vi "OP400ZP_SendToBddOP100ZENPlus.vi"(8 "errin":errorcluster, 11 "data in":string[](array[string])=["", "2022-08-23 16:19:54.000000", "0", "test base", "1.1", "2", "3", "4", "5", "6", "7", "8", "9", "10", "11", "12", "13", "14", "15", "16", "17", "18", "19", "20", "21", "22", "23", "24", "25", "26", "27", "1", "MOI", "28"]) -> (0 "error out":errorcluster, 3 "Chaîne":string)   [LabVIEW 2020]
uses:
  <vilib>/addons/database/Connection.llb/DB Tools Open Connec (String).vi
  <vilib>/addons/database/Connection.llb/Conn Execute.vi
  <vilib>/addons/database/Recordset.llb/Rec Destroy - Connection.vi
  <vilib>/addons/database/NI_Database_API.lvlib
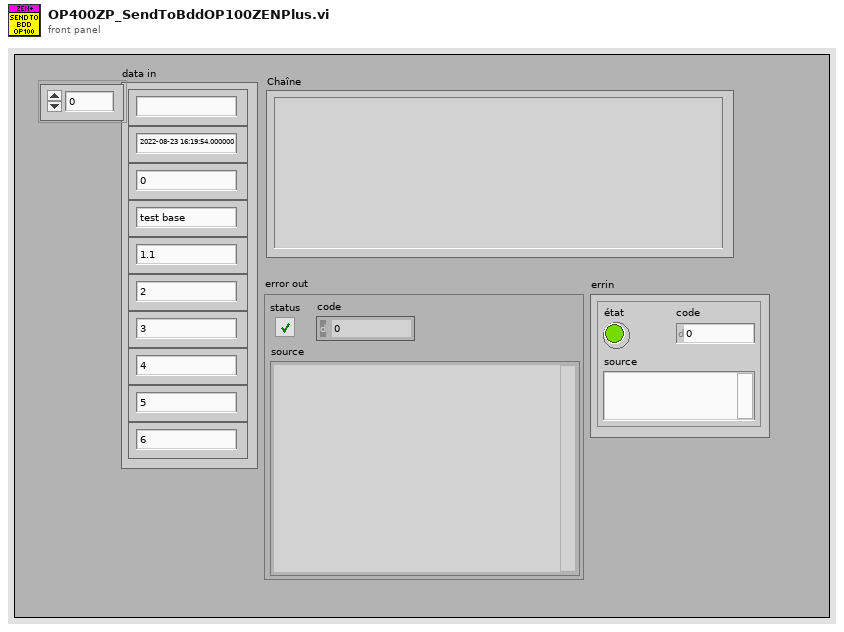
[diagram p1: front panel]
types:
  T1 = typedef "NI_Database_API.lvlib/Conn ObjectReference.ctl" = refnum<k1>
  T2 = typedef "NI_Database_API.lvlib/Rec ObjectReference.ctl" = refnum<k1>
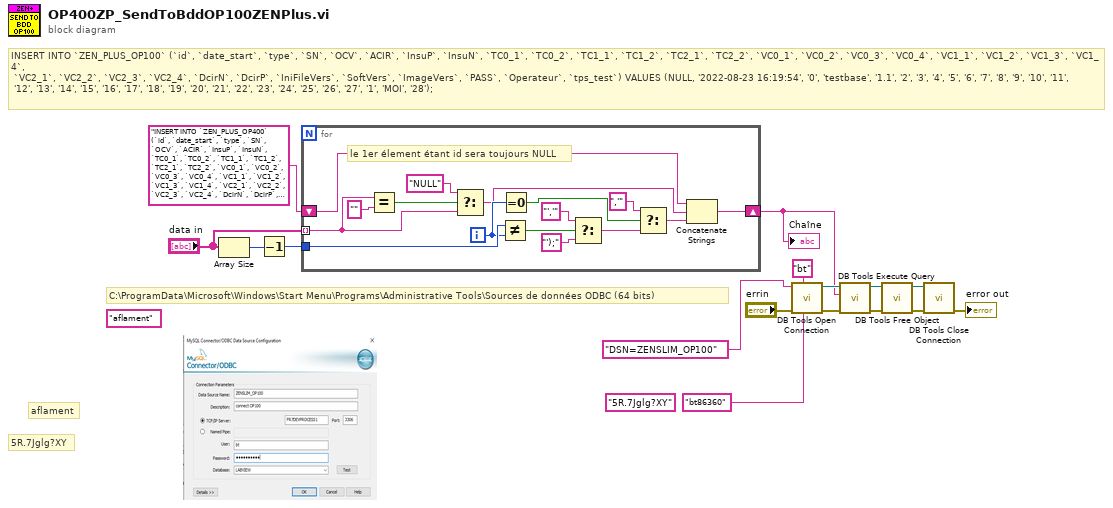
[diagram p0: block diagram]
diagram:
  (unwired) "aflament" ("userID")
  (unwired) "5R.7Jglg?XY" ("password")
  # "C:\\ProgramData\\Microsoft\\Windows\\Start Menu\\Programs\\Administrative Tools\\Sources de données ODBC (64 bits)"
  # "5R.7Jglg?XY"
  # "aflament"
  # "INSERT INTO `ZEN_PLUS_OP100` (`id`, `date_start`, `type`, `SN`, `OCV`, `ACIR`, `InsuP`, `InsuN`, `TC0_1`, `TC0_2`, `TC1_1`, `TC1_2`, `TC2_1`, `TC2_2`, `VC0_1`, `VC0_2`, `VC0_3`, `VC0_4`, `VC1_1`, `VC1_2`, `VC1_3`, `VC1_4`,\n `VC2_1`, `VC2_2`, `VC2_3`, `VC2_4`, `DcirN`, `DcirP`, `IniFileVers`, `SoftVers`, `ImageVers`, `PASS`, `Operateur`, `tps_test`) VALUES (NULL, '2022-08-23 16:19:54', '0', 'testbase', '1.1', '2', '3', '4', '5', '6', '7', '8', '9', '10', '11',\n '12', '13', '14', '15', '16', '17', '18', '19', '20', '21', '22', '23', '24', '25', '26', '27', '1', 'MOI', '28');"
  n1 = Array Size(array="data in") -> (size(s)=w15:i32)
  n2 = Decrement(x=w15) -> (x-1=w14:i32)
  n3 = for {
    tunnel: "data in" -> [w20] mode=indexing
    tunnel: w14 -> [w32]
    shift-right: [w28] -> w3
    shift-left: "INSERT INTO `ZEN_PLUS_OP400` (`id`, `date_start`, `type`, `SN`, `OCV`, `ACIR`, `InsuP`, `InsuN`, `TC0_1`, `TC0_2`, `TC1_1`, `TC1_2`, `TC2_1`, `TC2_2`, `VC0_1`, `VC0_2`, `VC0_3`, `VC0_4`, `VC1_1`, `VC1_2`, `VC1_3`, `VC1_4`, `VC2_1`, `VC2_2`, `VC2_3`, `VC2_4`, `DcirN`, `DcirP`, `IniFileVers`, `SoftVers`, `ImageVers`, `PASS`, `Operateur`, `tps_test`) VALUES (" -> [w29]
    i -> [w25]
    # "le 1er élement étant id sera toujours NULL"
    n4 = Equal?(x=w20, y="") -> (x = y?=w21:bool)
    n5 = Select(t="NULL" ("cas vrai"), s=w21, f=w20) -> (s? t:f=w18:string)
    n6 = Not Equal?(x=w32, y=w25) -> (x != y?=w31:bool)
    n7 = Equal To 0?(x=w25) -> (x = 0?=w26:bool)
    n8 = Select(t="','" ("chaîne"), s=w31, f="');" ("cas faux")) -> (s? t:f=w27:string)
    n9 = Select(t=",'" ("cas vrai"), s=w26, f=w27) -> (s? t:f=w23:string)
    n10 = Concatenate Strings(w29, w18, w23) -> (w28:string)
  }
  "Chaîne" <- w3
  n11 = call-poly <vilib>:"DB Tools Open Connection.vi"("password"="bt86360", "userID"="bt", "error in (no error)"="errin", "connection information"="DSN=ZENSLIM_OP100") -> ("error out"=w12:errorcluster, "connection reference"=w11:T1)  [unwired: 4 in]
  n12 = call-poly <vilib>:"DB Tools Execute Query.vi"("error in (no error)"=w12, "SQL query"=w3, "connection reference"=w11) -> ("error out"=w8:errorcluster, "recordset reference"=w7:T2)  [unwired: 5 in]
  n13 = call-poly <vilib>:"DB Tools Free Object.vi"("error in (no error)"=w8, "recordset reference"=w7) -> ("error out"=w9:errorcluster, "connection reference"=w10:T1)  [unwired: 8 in]
  n14 = call <vilib>:"DB Tools Close Connection.vi"("error in (no error)"=w9, "connection reference"=w10) -> ("error out"=→"error out":errorcluster)  [unwired: 5 in]
